vi "Read database.vi"(0 "condition":string="([数据标识] = 'N' or  [数据标识] = 'L') ", 1 "显示项":string[](array[string])=["top 100 *"], 5 "Table":string(combo)="CODMn", 7 "量程下拉列表":enum16{"低量程", "高量程"}(ring), 9 "量程筛选":bool, 11 "error in (no error)":errorcluster caption="错误输入（无错误）") -> (4 "表格":string[][](table), 6 "columns":string[](array[string]), 8 "foretime":string, 10 "lasttime":string, 15 "error out":errorcluster caption="错误输出")   [LabVIEW 2016, in "斯坦道CODMn.lvlib"]
uses:
  <vilib>/addons/database/Connection.llb/DB Tools Open Connec (String).vi
  <userlib>/_LVST/sqlite_api/Core/Tables/SQLite_List Columns.vi
  <vilib>/addons/database/_DB Variant To Data/Database Variant To Data.xnode
  <vilib>/addons/database/NI_Database_API.lvlib
  database/Access/Access Lib.lvlib
  database/SQLite/SQLite Lib.lvlib
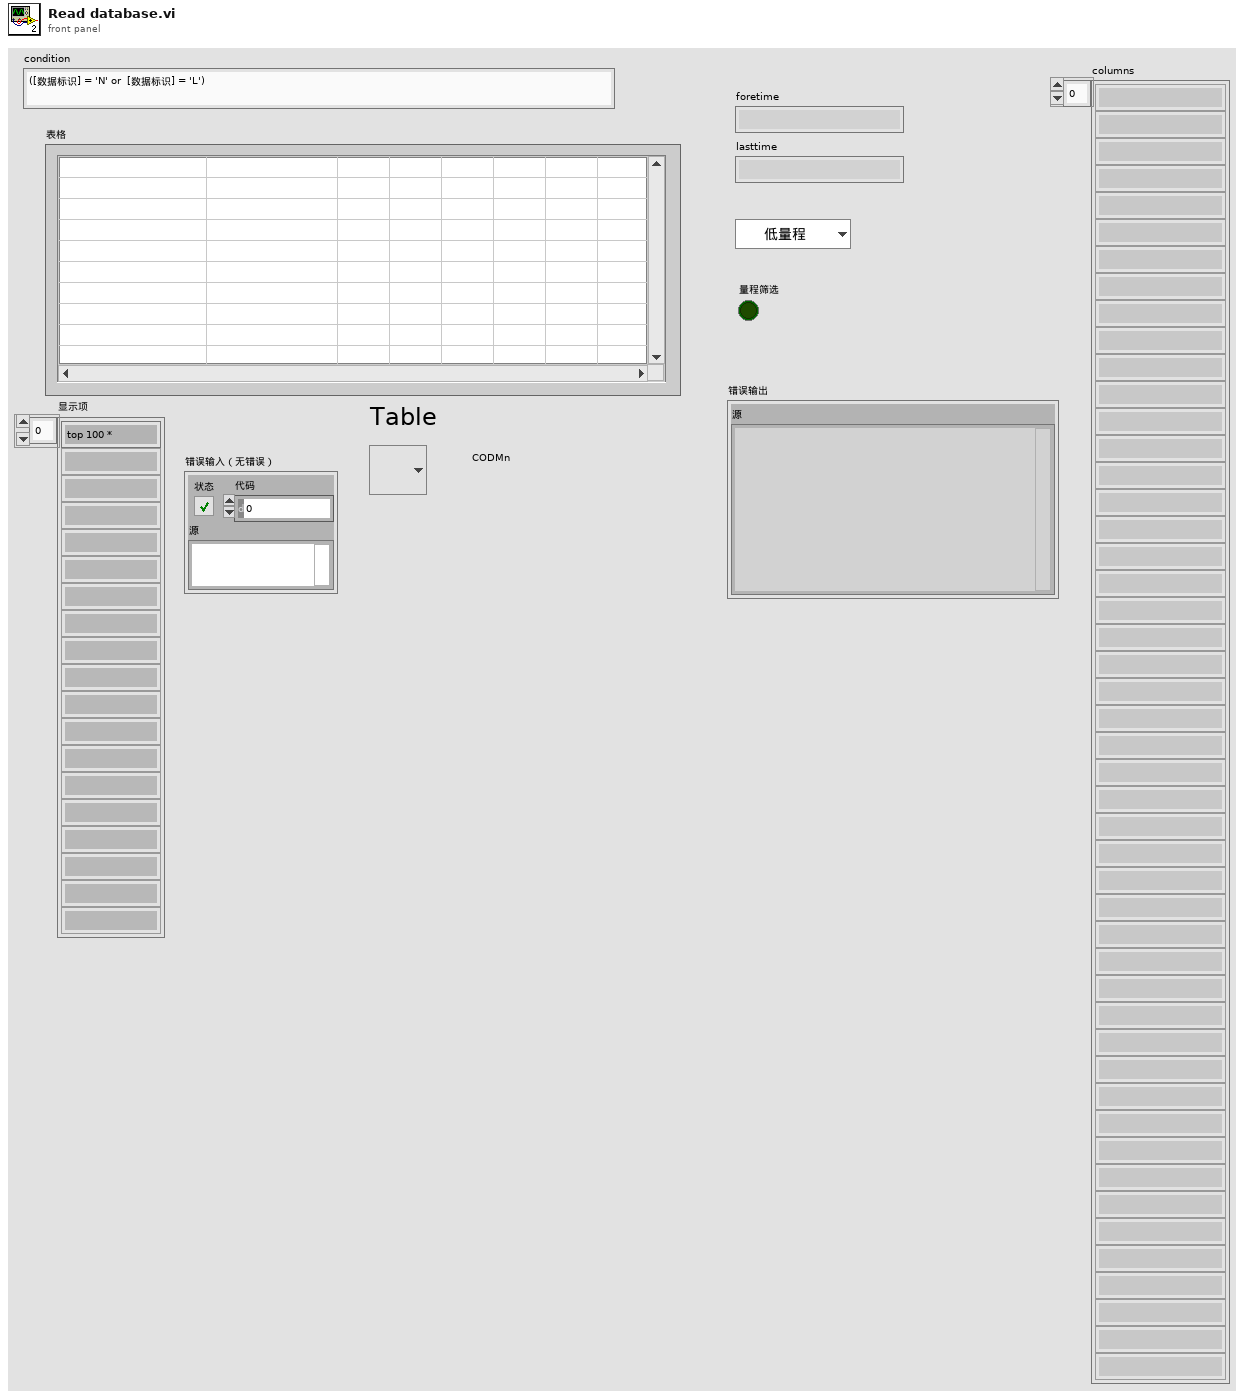
[diagram p1: front panel]
types:
  T1 = typedef "数据库类型.ctl" = enum16{"Access", "SQLite"}
  T2 = typedef "NI_Database_API.lvlib/Conn ObjectReference.ctl" = refnum<k1>
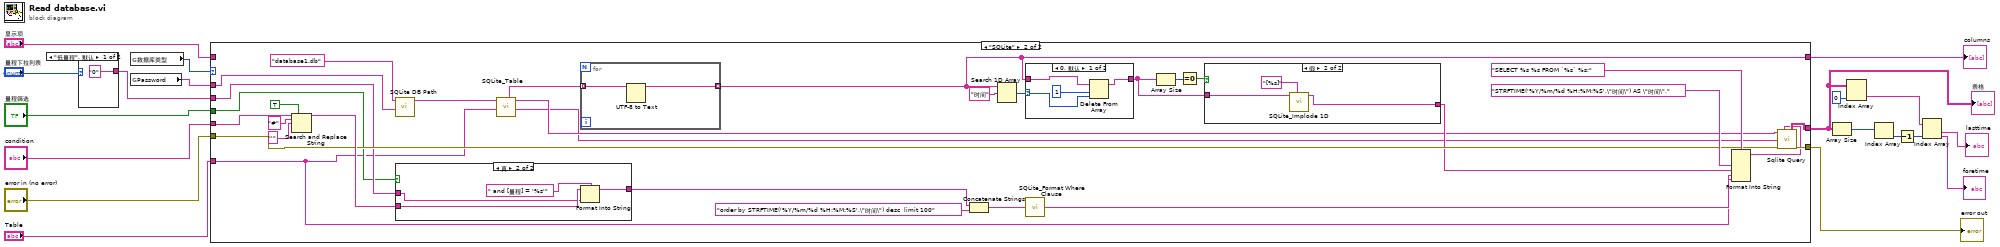
[diagram p0: block diagram]
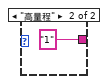
[diagram p2: hidden frame]
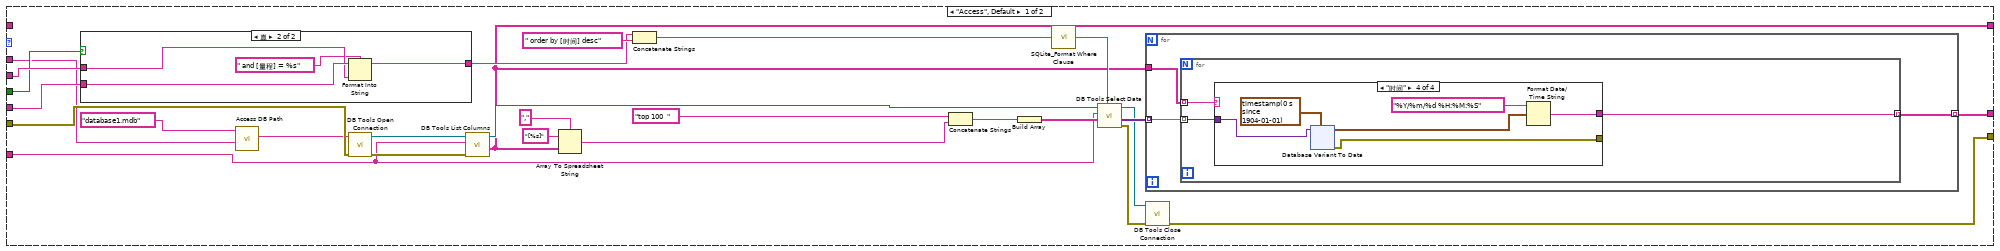
[diagram p3: hidden frame]
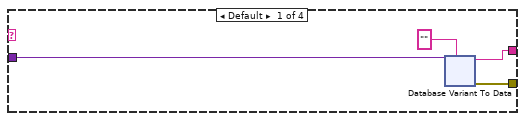
[diagram p5: hidden frame]
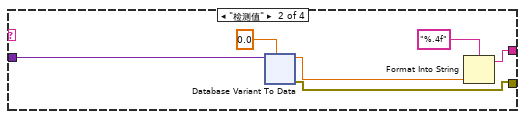
[diagram p6: hidden frame]
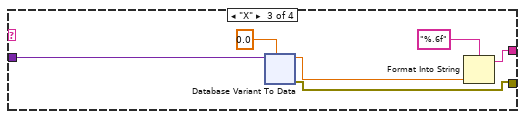
[diagram p7: hidden frame]
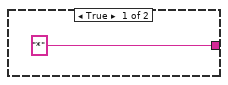
[diagram p10: hidden frame]
diagram:
  n1 = case shown="\"低量程\", 默认" "量程下拉列表" {
    tunnel: ["0" "1"] -> w5
    frame "低量程", Default {
    }
    frame "高量程" {
    }
  }
  n2 = global read "外部调用接口全局变量.vi" "数据库类型"() -> (w2:T1)
  n3 = global read "外部调用接口全局变量.vi" "Password"() -> (w1:string)
  n4 = case shown="\"SQLite\"" w2 {
    tunnel: "condition" -> [w29 w252]
    tunnel: "显示项" -> [_ _]
    tunnel: "Table" -> [w25 w227]
    tunnel: "error in (no error)" -> [w43 w239]
    tunnel: [w35 w238] -> w17
    tunnel: [w34 w234] -> w11
    tunnel: w5 -> [w31 w232]
    tunnel: "量程筛选" -> [w30 w230]
    tunnel: [w23 w224] -> w3
    tunnel: w1 -> [w22 w223]
    frame "Access", Default {
      n5 = case shown="真" w30 {
        tunnel: w29 -> [w49 w53]
        tunnel: [w49 w52] -> w32
        tunnel: w31 -> [_ w51]
        frame False {
        }
        frame True {
          n6 = Format Into String(format string=" and [量程] = %s" ("格式字符串"), initial string=w53, w51) -> (resulting string=w52:string)  [unwired: 1 in, 1 out]
        }
      }
      n7 = call "Access DB Path.vi"("Password"=w22, "database"="database1.mdb") -> ("Connection information"=w28:string)  [unwired: 8 in, 1 out]
      n8 = call-poly <vilib>:"DB Tools Open Connection.vi"("error in (no error)"=w43, "connection information"=w28) -> ("error out"=w26:errorcluster, "connection reference"=w27:T2)  [unwired: 6 in]
      n9 = call <vilib>:"DB Tools List Columns.vi"("error in (no error)"=w26, "table"=w25, "connection reference"=w27) -> ("columns"=w23:string[], "connection reference out"=w24:T2)  [unwired: 1 in, 2 out]
      n10 = Array To Spreadsheet String(delimiter (Tab)="," ("分隔符(Tab)"), array=w23, 3:"[%s]" ("格式字符串")) -> (spreadsheet string=w41:string)
      n11 = Concatenate Strings(w32, " order by [时间] desc" ("字符串")) -> (w47:string)
      n12 = Concatenate Strings("top 100  " ("字符串"), w41) -> (w40:string)
      n13 = Build Array(w40) -> (w39:string[])
      n14 = call <userlib>:"SQLite_Format Where Clause.vi"("Where clause"=w47) -> ("String"=w33:string)  [unwired: 4 in]
      n15 = call <vilib>:"DB Tools Select Data.vi"("condition"=w33, "columns"=w39, "table"=w25, "connection reference"=w24) -> ("error out"=w36:errorcluster, "data"=w38:variant[][], "connection reference out"=w37:T2)  [unwired: 2 in]
      n16 = for {
        tunnel: w38 -> [w56] mode=indexing
        tunnel: [w55] -> w34 mode=indexing
        tunnel: w23 -> [w54]
        n17 = for {
          tunnel: w56 -> [w58] mode=indexing
          tunnel: [w59] -> w55 mode=indexing
          tunnel: w54 -> [w57] mode=indexing
          n18 = case shown="\"时间\"" w57 {
            tunnel: w58 -> [w63 w101 w139 w177]
            tunnel: [w60 w97 w135 w173] -> w59
            tunnel: [w61 w100 w138 w172] -> _
            frame Default {
              n19 = xnode "Database Variant To Data"("database variant"=w63, "type"="") -> ("data"=w60:string, "error out"=w61:errorcluster)  [unwired: 1 in]
            }
            frame "检测值" {
              n20 = xnode "Database Variant To Data"("database variant"=w101, "type"=0.0) -> ("data"=w98:dbl, "error out"=w100:errorcluster)  [unwired: 1 in]
              n21 = Format Into String(format string="%.4f" ("格式字符串"), w98) -> (resulting string=w97:string)  [unwired: 2 in, 1 out]
            }
            frame "X" {
              n22 = xnode "Database Variant To Data"("database variant"=w139, "type"=0.0) -> ("data"=w136:dbl, "error out"=w138:errorcluster)  [unwired: 1 in]
              n23 = Format Into String(format string="%.6f" ("格式字符串"), w136) -> (resulting string=w135:string)  [unwired: 2 in, 1 out]
            }
            frame "时间" {
              n24 = xnode "Database Variant To Data"("database variant"=w177, "type"=timestamp(0 s since 1904-01-01) ("当前时间")) -> ("data"=w176:timestamp, "error out"=w172:errorcluster)  [unwired: 1 in]
              n25 = Format Date/Time String(time format string (%c)="%Y/%m/%d %H:%M:%S" ("时间格式字符串(%c)"), seconds (now)=w176) -> (date/time string=w173:string)  [unwired: 1 in]
            }
          }
        }
      }
      n26 = call <vilib>:"DB Tools Close Connection.vi"("error in (no error)"=w36, "connection reference"=w37) -> ("error out"=w35:errorcluster)  [unwired: 5 in]
    }
    frame "SQLite" {
      n27 = Search and Replace String(replace all?=TRUE ("替换全部？(F)"), input string=w252, search string="#" ("搜索字符串"), replace string="'" ("替换字符串(\"\")")) -> (result string=w241:string)  [unwired: 4 in, 3 out]
      n28 = call "SQLite DB Path.vi"("Password"=w223, "database"="database1.db") -> ("Path out"=w229:string)  [unwired: 9 in]
      n29 = case shown="真" w230 {
        tunnel: w241 -> [w256 w260]
        tunnel: [w256 w259] -> w233
        tunnel: w232 -> [_ w257]
        frame False {
        }
        frame True {
          n30 = Format Into String(format string=" and [量程] = '%s'" ("格式字符串"), initial string=w260, w257) -> (resulting string=w259:string)  [unwired: 1 in, 1 out]
        }
      }
      n31 = call-poly <userlib>:"SQLite_Table.vi"("DB Path"=w229, "Table Name"=w227) -> ("Columns"=w226:string[], "DB Path Out"=w228:string, "Table Name Out"=w225:string)  [unwired: 5 in, 1 out]
      n32 = for {
        tunnel: w226 -> [w255] mode=indexing
        tunnel: [w254] -> w224 mode=indexing
        n33 = UTF-8 to Text(11:w255) -> (3:w254:string)  [unwired: 2 in, 1 out]
      }
      n34 = Concatenate Strings(w233, "order by STRFTIME('%Y/%m/%d %H:%M:%S',\"时间\") desc  limit 100") -> (w237:string)
      n35 = Search 1D Array(1D array=w224, element="时间" ("元素")) -> (index of element=w245:i32)  [unwired: 1 in]
      n36 = case shown="0, 默认" w245 {
        selector: w245 -> [w263 _]
        tunnel: w224 -> [w264 w265]
        tunnel: [w261 w265] -> w246
        frame 0, Default {
          n37 = Delete From Array(array=w264, length=1 ("长度"), index=w263) -> (array with subset deleted=w261:string[])  [unwired: 1 out]
        }
        frame -1 {
        }
      }
      n38 = call <userlib>:"SQLite_Format Where Clause.vi"("Where clause"=w237) -> ("String"=w236:string)  [unwired: 4 in]
      n39 = Array Size(array=w246) -> (size(s)=w242:i32)
      n40 = Equal To 0?(x=w242) -> (x = 0?=w243:bool)
      n41 = case shown="假" w243 {
        tunnel: w246 -> [_ w268]
        tunnel: ["*" ("t") w267] -> w235
        frame True {
        }
        frame False {
          n42 = call <userlib>:"SQLite_Implode 1D.vi"("Values"=w268, "format string"="[%s]") -> ("imploded string"=w267:string)  [unwired: 7 in, 1 out]
        }
      }
      n43 = Format Into String(format string="SELECT %s %s FROM `%s` %s;" ("SQL Query"), "STRFTIME('%Y/%m/%d %H:%M:%S',\"时间\") AS \"时间\",", w235, w227, w236) -> (resulting string=w231:string)  [unwired: 2 in, 1 out]
      n44 = call "Sqlite Query.vi"("DB Path"=w228, "SQL Query"=w231, "Tables Name"=w225, "error in (no error)"=w239) -> ("Results"=w234:string[][], "error out"=w238:errorcluster)  [unwired: 9 in, 1 out]
    }
  }
  "表格" <- w11
  "error out" <- w17
  "columns" <- w3
  n45 = Array Size(array=w11) -> (size(s)=w14:i32[])
  n46 = Index Array(array=w11, index (col)=0 ("禁用的索引 (列)")) -> (element=w15:string[])  [unwired: 1 in]
  n47 = Index Array(array=w14) -> (element=w13:i32)  [unwired: 1 in]
  n48 = Decrement(x=w13) -> (x-1=w12:i32)
  n49 = Index Array(array=w15, index #2=w12) -> (element #1=→"lasttime":string, element #2=→"foretime":string)  [unwired: 1 in]
